vi "Test Withdraw Successful When Emptying Account.vi"(8 "error in (no error)":errorcluster, 11 "Test Case In":refnum<class "Controller Test.lvclass">) -> (0 "error out":errorcluster, 3 "Test Case Out":refnum<class "Controller Test.lvclass">)   [LabVIEW 2020, in "Controller Test.lvclass"]
uses:
  Controller Test/Controller Test.lvclass
  C:/Program Files (x86)/National Instruments/LabVIEW 2020/vi.lib/Astemes/LUnit/Test Case.lvclass
  Account Database/Account Data.ctl
  ATM Controller/State.ctl
  <vilib>/Astemes/LUnit/Test Case.lvclass/Test Case.ctl
  01074fa8-ee8a-411d-bc8b-fc92c4f90959.vi
  <vilib>/Astemes/LUnit/Palette/Pass.vi
  <vilib>/Astemes/LUnit/Palette/Fail.vi
  <vilib>/Astemes/LUnit/Compare Variants.vi
  <vilib>/Astemes/LUnit/Describe Comparison.vi
  <vilib>/Astemes/LUnit/Set Assertion Type.vi
  <vilib>/Astemes/LUnit/Add test result.vi
  <vilib>/Astemes/LUnit/Variant to string.vi
  <vilib>/Astemes/LUnit/LUnit Record Assertion Result.vi
  <vilib>/Astemes/LUnit/LUnit Aggregate Assertion Results.vi
  <vilib>/Astemes/LUnit/Method Result/LUnit Merge Status.vi
  <vilib>/Astemes/LUnit/LUnit Concatenate result strings.vi
  <vilib>/Utility/Data Type/Get Type Information.vi
  <vilib>/Utility/LVClass/Get LV Class Name.vi
  Controller Test/Controller Test.lvclass/Controller Test.ctl
  ATM Controller/ATM Controller.lvclass
  Account Database/Account Database.lvclass
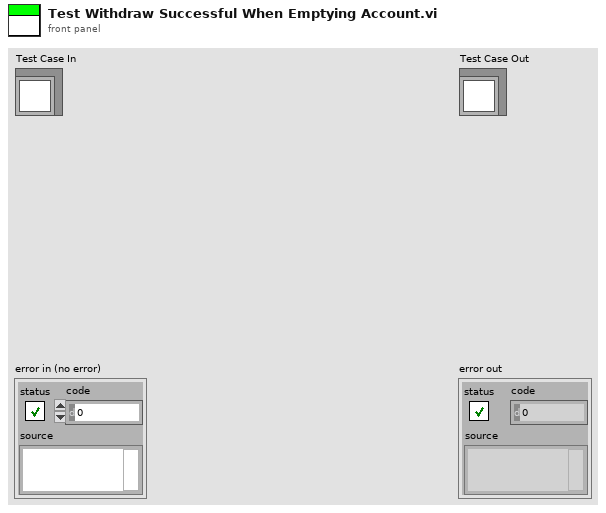
[diagram p1: front panel]
types:
  T1 = typedef "ATM Controller.lvclass/State.ctl" = enum16{"Start", "Card Inserted", "Verification Failed", "Verification Succeeded", "Depositing", "Depositing Completed", "Withdrawing", "Withdraw Completed", "Withdraw Failed", "Balance Inquiry", "Terminate"}
  T2 = typedef "Account Database.lvclass/Account Data.ctl" = cluster{"Account Number":string, "First Name":string, "Last Name":string, "Account Balance":string}
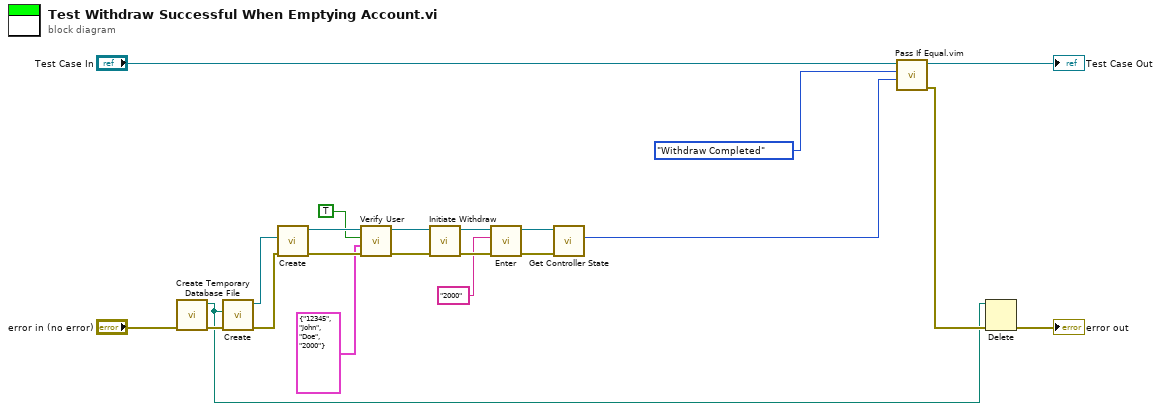
[diagram p0: block diagram]
diagram:
  n1 = call "Create Temporary Database File.vi"("error in (no error)"="error in (no error)") -> ("error out"=w7:errorcluster, "path"=w1:path)  [unwired: 9 in]
  n2 = call "Create.vi"("error in (no error)"=w7, "Data File"=w1) -> ("error out"=w6:errorcluster, "Account Database out"=w5:refnum<class "Account Database.lvclass">)  [unwired: 8 in]
  n3 = call "Create.vi"("error in (no error)"=w6, "Account Database"=w5) -> ("error out"=w18:errorcluster, "ATM Controller out"=w16:refnum<class "ATM Controller.lvclass">)  [unwired: 8 in]
  n4 = call "Verify User.vi"("error in (no error)"=w18, "Account Data"=T2 {"Account Number"="12345", "First Name"="John", "Last Name"="Doe", "Account Balance"="2000"}, "Verified?"=TRUE, "ATM Controller in"=w16) -> ("error out"=w17:errorcluster, "ATM Controller out"=w12:refnum<class "ATM Controller.lvclass">)  [unwired: 6 in]
  n5 = call "Initiate Withdraw.vi"("error in (no error)"=w17, "ATM Controller in"=w12) -> ("error out"=w13:errorcluster, "ATM Controller out"=w10:refnum<class "ATM Controller.lvclass">)  [unwired: 8 in]
  n6 = call "Enter.vi"("error in (no error)"=w13, "User Input"="2000", "ATM Controller in"=w10) -> ("error out"=w11:errorcluster, "ATM Controller out"=w9:refnum<class "ATM Controller.lvclass">)  [unwired: 7 in]
  n7 = call "Get Controller State.vi"("error in (no error)"=w11, "ATM Controller in"=w9) -> ("ATM State"=w4:T1)  [unwired: 7 in, 2 out]
  n8 = call "Pass If Equal.vim"("Actual"=w4, "Expected"=State."Withdraw Completed" ("ATM State"), "LUnit Test Case In"="Test Case In") -> ("error out"=w20:errorcluster, "LUnit Test Case Out"=→"Test Case Out":refnum<class "Controller Test.lvclass">)  [unwired: 7 in]
  n9 = Delete(path (use dialog)=w1, error in=w20) -> (error out=→"error out":errorcluster)  [unwired: 3 in, 2 out]
